vi "AlarmQueryRulesResponse_Create.vi"(7 "Header":T8, 8 "error in (no error)":errorcluster, 9 "ResponseError":errorcluster, 10 "AlarmQueryRulesResponse":T1, 11 "IRoutingSource":T7) -> (0 "error out":errorcluster, 3 "Message":T9)   [LabVIEW 2017]
uses:
  <vilib>/addons/InsightCM/MessageBus/Base/controls/Message.ctl
  <vilib>/addons/InsightCM/MessageBus/Base/controls/MessageHeader.ctl
  <vilib>/addons/InsightCM/MessageBus/Base/controls/KeyValuePair.ctl
  <vilib>/addons/InsightCM/MessageBus/Base/controls/IRoutingSource.ctl
  <vilib>/addons/InsightCM/MessageBus/MessageLibrary/Alarm/controls/AlarmQueryRulesResponseBody.ctl
  <vilib>/addons/InsightCM/MessageBus/Base/controls/AlarmRule.ctl
  <vilib>/addons/InsightCM/MessageBus/Base/controls/AlarmTrigger.ctl
  <vilib>/addons/InsightCM/MessageBus/Base/controls/AlarmCondition.ctl
  <vilib>/addons/InsightCM/MessageBus/Base/controls/AlarmAction.ctl
  <vilib>/addons/InsightCM/MessageBus/Base/controls/MessageClassType.ctl
  <vilib>/addons/InsightCM/Utilities/PropertyHelpers/PropertyHelpers.lvlib
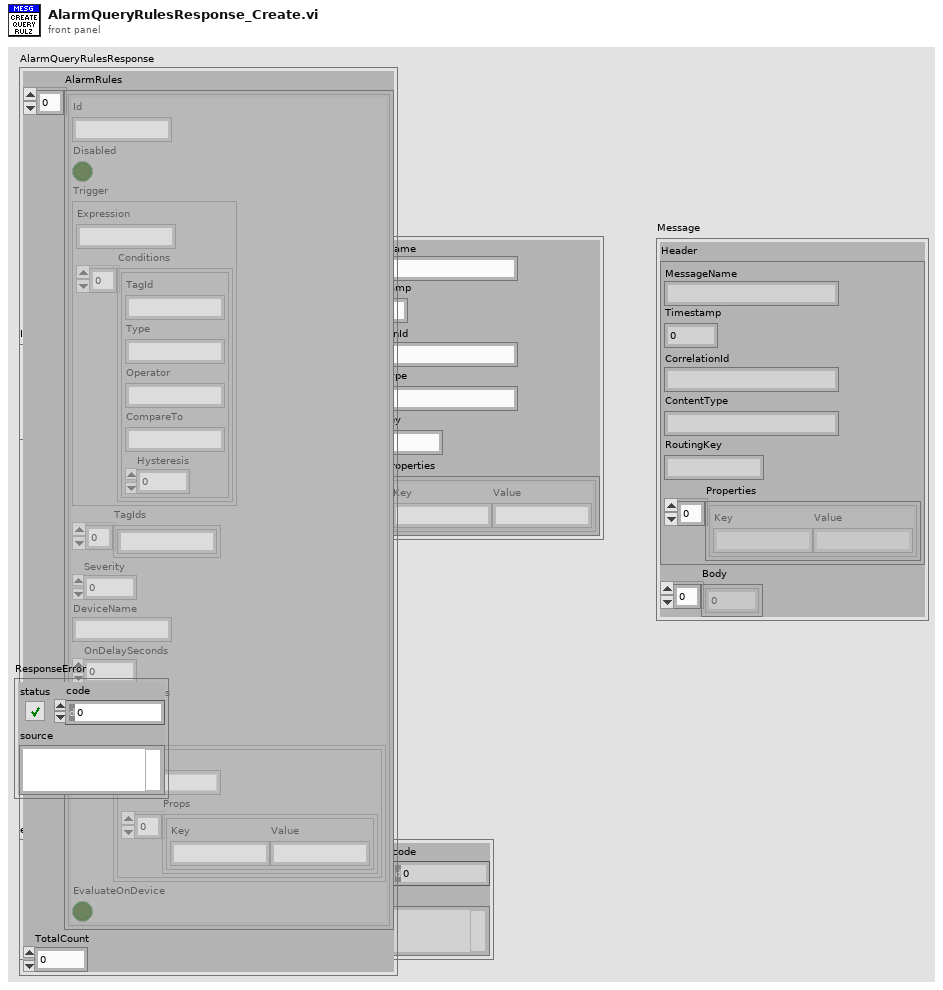
[diagram p1: front panel]
types:
  T1 = typedef "AlarmQueryRulesResponseBody.ctl" = cluster{"AlarmRules":T2[], "TotalCount":i32}
  T2 = typedef "AlarmRule.ctl" = cluster{"Id":string, "Disabled":bool, "Trigger":T3, "TagIds":string[], "Severity":i32, "DeviceName":string, "OnDelaySeconds":dbl, "OffDelaySeconds":dbl, "Actions":T5[], "EvaluateOnDevice":bool}
  T3 = typedef "AlarmTrigger.ctl" = cluster{"Expression":string, "Conditions":T4[]}
  T4 = typedef "AlarmCondition.ctl" = cluster{"TagId":string, "Type":string, "Operator":string, "CompareTo":string, "Hysteresis":dbl}
  T5 = typedef "AlarmAction.ctl" = cluster{"Type":string, "Props":T6[]}
  T6 = typedef "KeyValuePair.ctl" = cluster{"Key":string, "Value":string}
  T7 = typedef "IRoutingSource.ctl" = cluster{"CorrelationId":string, "ReplyTo":string}
  T8 = typedef "MessageHeader.ctl" = cluster{"MessageName":string, "Timestamp":i64, "CorrelationId":string, "ContentType":string, "RoutingKey":string, "Properties":T6[]}
  T9 = typedef "Message.ctl" = cluster{"Header":T8, "Body":u8[]}
  T10 = typedef "MessageClassType.ctl" = enum16{"Request", "Response", "Broadcast", "RoutedMessage"}
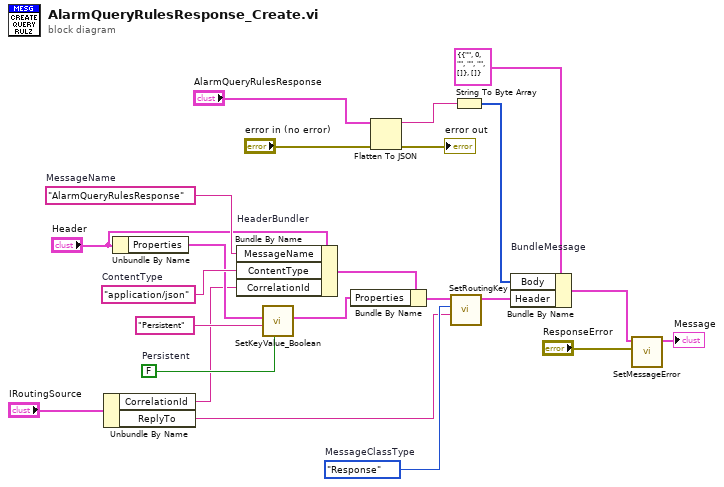
[diagram p0: block diagram]
diagram:
  w19 = MessageClassType."Response"  # MessageClassType
  w14 = FALSE  # Persistent
  w20 = "AlarmQueryRulesResponse"  # MessageName
  w17 = "application/json"  # ContentType
  n1 = Unbundle By Name("IRoutingSource") -> ("CorrelationId"=w4:string, "ReplyTo"=w3:string)
  n2 = Unbundle By Name("Header") -> ("Properties"=w16:T6[])
  n3 = Bundle By Name "HeaderBundler"(cluster="Header", "MessageName"=w20, "ContentType"=w17, "CorrelationId"=w4) -> (w11:T8)
  n4 = call <vilib>:"SetKeyValue_Boolean.vi"("value"=w14, "key"="Persistent" ("Key"), "key value pairs"=w16) -> ("key value pairs out"=w10:T6[])  [unwired: 8 in]
  n5 = Bundle By Name(cluster=w11, "Properties"=w10) -> (w12:T8)
  n6 = Flatten To JSON(anything="AlarmQueryRulesResponse", error in (no error)="error in (no error)") -> (JSON string=w2:string, 11:→"error out":errorcluster)  [unwired: 1 in]
  n7 = call <vilib>:"SetRoutingKey.vi"("SendTo"=w3, "MessageClassType"=w19, "Message Header in"=w12) -> ("Message Header out"=w13:T8)  [unwired: 8 in]
  n8 = String To Byte Array(string=w2) -> (unsigned byte array=w22:u8[])
  n9 = Bundle By Name "BundleMessage"(cluster=T9 {"Header"={"MessageName"="", "Timestamp"=0, "CorrelationId"="", "ContentType"="", "RoutingKey"="", "Properties"=[]}, "Body"=[]} ("Message"), "Body"=w22, "Header"=w13) -> (w8:T9)
  n10 = call <vilib>:"SetMessageError.vi"("error"="ResponseError", "message in"=w8) -> ("message out"=→"Message":T9)  [unwired: 9 in]
